vi "高温报警流程.vi"   [LabVIEW 2016]
uses:
  PLC/PLC.lvlib
types:
  T1 = enum16{"报警状态监测", "报警确认", "仪器断电", "市电断电", "工控机关机", "取消告警", "结束"}
  T2 = cluster{"时间标识":timestamp, "设备":string, "日志信息":string, "备注":string}
  T3 = cluster{"时间标识":timestamp, "设备":string, "日志信息":string, "流程参数":string}
  T4 = cluster{"AD0":sgl, "AD1":sgl, "AD2":sgl, "AD3":sgl, "AD4":sgl, "AD5":sgl}
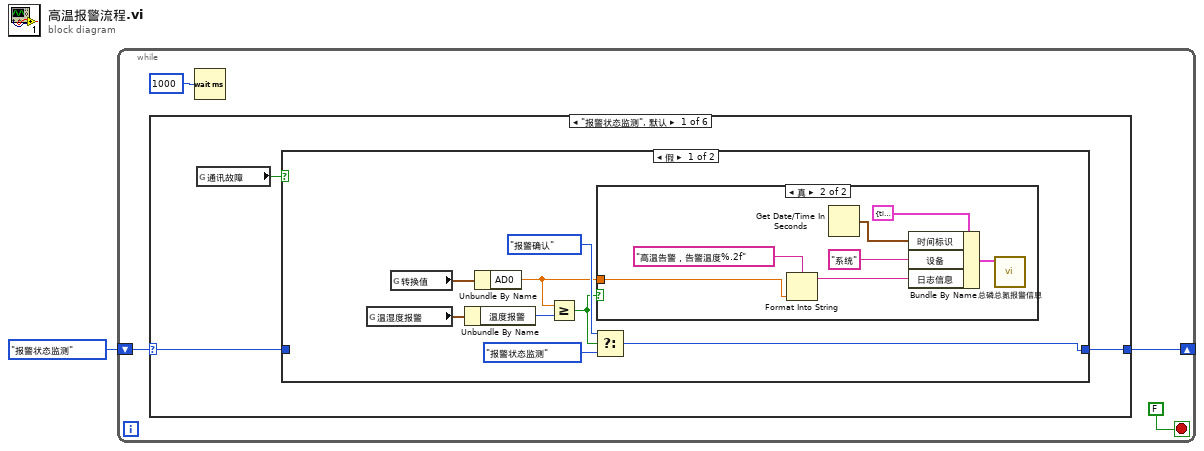
[diagram p0: block diagram]
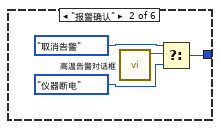
[diagram p4: hidden frame]
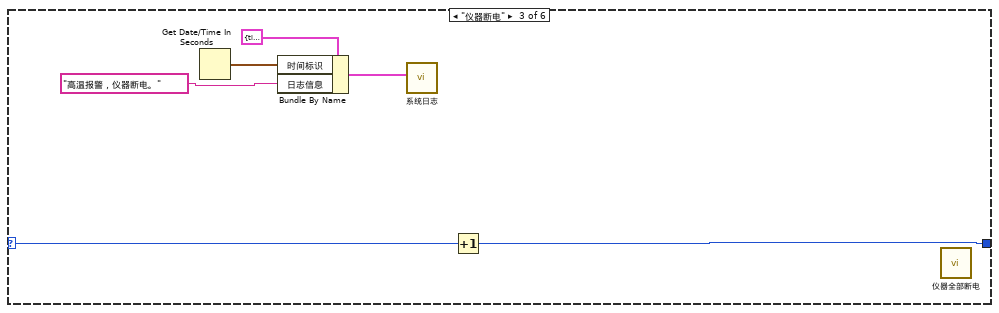
[diagram p5: hidden frame]
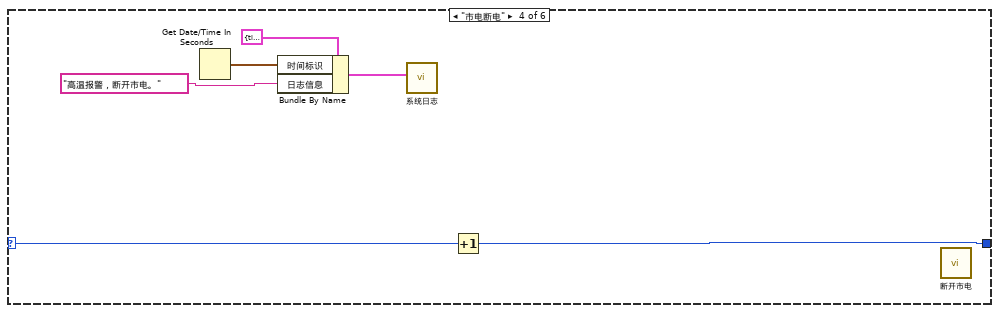
[diagram p6: hidden frame]
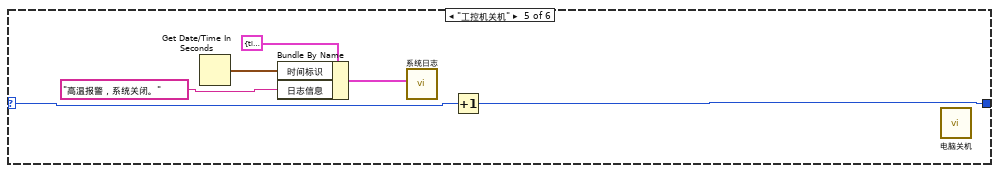
[diagram p7: hidden frame]
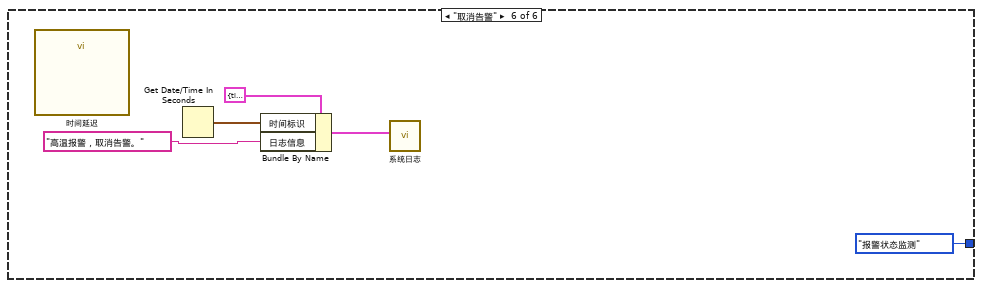
[diagram p8: hidden frame]
diagram:
  n1 = while {
    shift-right: [w3] -> _
    shift-left: T1."报警状态监测" ("枚举") -> [w4]
    stop <- FALSE stop-if-true
    n2 = case shown="\"报警状态监测\", 默认" w4 {
      selector: w4 -> [w6 _ w34 w40 w46 _]
      tunnel: [w8 w27 w33 w39 w45 T1."报警状态监测" ("枚举")] -> w3
      frame "报警状态监测", Default {
        n3 = global read "采配水全局变量.vi" "通讯故障"() -> (w7:bool)
        n4 = case shown="假" w7 {
          tunnel: [w13 w24] -> w8
          tunnel: w6 -> [_ w24]
          frame False {
            n5 = global read "系统设置全局变量.vi" "温湿度报警"() -> (w15:cluster{"温度报警":u16, "湿度报警":u16, "报警确认时间":u16})
            n6 = global read "采配水全局变量.vi" "转换值"() -> (w16:T4)
            n7 = Unbundle By Name(w15) -> ("温度报警"=w14:u16)
            n8 = Unbundle By Name(w16) -> ("AD0"=w9:sgl)
            n9 = Greater Or Equal?(x=w9, y=w14) -> (x >= y?=w10:bool)
            n10 = Select(t=T1."报警确认" ("枚举"), s=w10, f=T1."报警状态监测" ("枚举")) -> (s? t:f=w13:T1)
            n11 = case shown="真" w10 {
              tunnel: w9 -> [_ w19]
              frame False {
              }
              frame True {
                n12 = Format Into String(format string="高温告警，告警温度%.2f" ("格式字符串"), w19) -> (resulting string=w17:string)  [unwired: 2 in, 1 out]
                n13 = Get Date/Time In Seconds() -> (seconds since 1Jan1904=w22:timestamp)
                n14 = Bundle By Name(cluster=T2 {"时间标识"=timestamp(0 s since 1904-01-01), "设备"="", "日志信息"="", "备注"=""} ("data in"), "时间标识"=w22, "设备"="系统", "日志信息"=w17) -> (w21:T2)
                n15 = call "总磷总氮报警信息.vi"("data in"=w21) -> ()  [unwired: 10 in, 1 out]
              }
            }
          }
          frame True {
          }
        }
      }
      frame "报警确认" {
        n16 = call "高温告警对话框.vi"() -> ("T button?"=w28:bool)  [unwired: 11 in]
        n17 = Select(t=T1."取消告警" ("枚举"), s=w28, f=T1."仪器断电" ("枚举")) -> (s? t:f=w27:T1)
      }
      frame "仪器断电" {
        n18 = Get Date/Time In Seconds() -> (seconds since 1Jan1904=w31:timestamp)
        n19 = Bundle By Name(cluster=T3 {"时间标识"=timestamp(0 s since 1904-01-01), "设备"="系统", "日志信息"="", "流程参数"=""} ("data in"), "时间标识"=w31, "日志信息"="高温报警，仪器断电。") -> (w30:T3)
        n20 = call "系统日志.vi"("data in"=w30) -> ()  [unwired: 11 in]
        n21 = Increment(x=w34) -> (x+1=w33:T1)
        n22 = call "仪器全部断电.vi"() -> ()  [unwired: 12 in]
      }
      frame "市电断电" {
        n23 = Get Date/Time In Seconds() -> (seconds since 1Jan1904=w37:timestamp)
        n24 = Bundle By Name(cluster=T3 {"时间标识"=timestamp(0 s since 1904-01-01), "设备"="系统", "日志信息"="", "流程参数"=""} ("data in"), "时间标识"=w37, "日志信息"="高温报警，断开市电。") -> (w36:T3)
        n25 = call "系统日志.vi"("data in"=w36) -> ()  [unwired: 11 in]
        n26 = Increment(x=w40) -> (x+1=w39:T1)
        n27 = call "断开市电.vi"() -> ()  [unwired: 12 in]
      }
      frame "工控机关机" {
        n28 = Get Date/Time In Seconds() -> (seconds since 1Jan1904=w43:timestamp)
        n29 = Bundle By Name(cluster=T3 {"时间标识"=timestamp(0 s since 1904-01-01), "设备"="系统", "日志信息"="", "流程参数"=""} ("data in"), "时间标识"=w43, "日志信息"="高温报警，系统关闭。") -> (w42:T3)
        n30 = call "系统日志.vi"("data in"=w42) -> ()  [unwired: 11 in]
        n31 = Increment(x=w46) -> (x+1=w45:T1)
        n32 = call "电脑关机.vi"() -> ()  [unwired: 12 in]
      }
      frame "取消告警" {
        n33 = call "时间延迟"() -> ()  [unwired: 11 in, 1 out]
        n34 = Get Date/Time In Seconds() -> (seconds since 1Jan1904=w49:timestamp)
        n35 = Bundle By Name(cluster=T3 {"时间标识"=timestamp(0 s since 1904-01-01), "设备"="系统", "日志信息"="", "流程参数"=""} ("data in"), "时间标识"=w49, "日志信息"="高温报警，取消告警。") -> (w48:T3)
        n36 = call "系统日志.vi"("data in"=w48) -> ()  [unwired: 11 in]
      }
    }
    n37 = Wait (ms)(milliseconds to wait=u32 1000 ("等待时间（毫秒）")) -> ()  [unwired: 1 out]
  }
